vi "LatchClose.vi"   [LabVIEW 2014, in "LatchLib.lvlib"]
uses:
  LatchLib.lvlib
  LatchRefs.ctl
types:
  T1 = typedef "LatchLib.lvlib/LatchRefs.ctl" = enum16{"LatchSloenoid", "ContainerSolenoid"}
  T2 = typedef "WPI_SolenoidDevRef.ctl" = cluster{"DevStatus":errorcluster, "Pneumatics Control Module":u8, "Forward Solenoid Channel":T3, "Reverse Solenoid Channel":T3}
  T3 = typedef "WPI_SolenoidChannel.ctl" = enum8{"Solenoid 0", "Solenoid 1", "Solenoid 2", "Solenoid 3", "Solenoid 4", "Solenoid 5", "Solenoid 6", "Solenoid 7", "Invalid"}
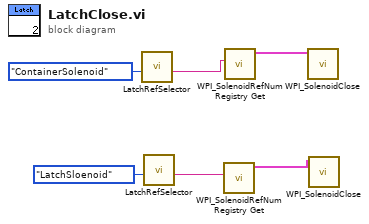
[diagram p0: block diagram]
diagram:
  n1 = call "LatchRefSelector.vi"("Enum"=LatchRefs."ContainerSolenoid") -> ("String"=w2:string)  [unwired: 10 in]
  n2 = call "LatchRefSelector.vi"("Enum"=LatchRefs."LatchSloenoid") -> ("String"=w3:string)  [unwired: 10 in]
  n3 = call <vilib>:"WPI_SolenoidRefNum Registry Get.vi"("refnum name"=w3) -> ("SolenoidDevRef"=w6:T2)  [unwired: 9 in, 1 out]
  n4 = call <vilib>:"WPI_SolenoidRefNum Registry Get.vi"("refnum name"=w2) -> ("SolenoidDevRef"=w1:T2)  [unwired: 9 in, 1 out]
  n5 = call <vilib>:"WPI_SolenoidClose.vi"("SolenoidDevRef"=w1) -> ()  [unwired: 10 in, 1 out]
  n6 = call <vilib>:"WPI_SolenoidClose.vi"("SolenoidDevRef"=w6) -> ()  [unwired: 10 in, 1 out]
